vi "Add Record.vi"(8 "Error In (no error)":errorcluster, 10 "Data":variant, 11 "DB Operator in":refnum<class "DB Operator.lvclass">) -> (0 "Error Out":errorcluster, 3 "DB Operator out":refnum<class "DB Operator.lvclass">)   [LabVIEW 2023, in "DB Operator.lvclass"]
uses:
  DB Operator.lvclass
  Ctrls/DB Controls/Category.ctl
  Ctrls/DB Controls/Cycle.ctl
  Ctrls/DB Controls/Saving Goal.ctl
  Ctrls/DB Controls/Saving.ctl
  Ctrls/DB Controls/Subcategory.ctl
  Ctrls/DB Controls/Transaction.ctl
  DB Operator.lvclass/DB Operator.ctl
  <vilib>/Utility/Data Type/NI_Data Type.lvlib
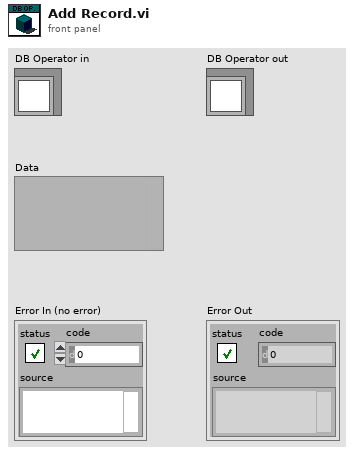
[diagram p1: front panel]
types:
  T1 = typedef "DB Operator.lvclass/Category.ctl" = cluster{"ID":u32, "Name":string}
  T2 = typedef "DB Operator.lvclass/Cycle.ctl" = cluster{"ID":u32, "Name":string, "Day of Month":u8, "Description":string}
  T3 = typedef "DB Operator.lvclass/Saving Goal.ctl" = cluster{"ID":u64, "Is Active":bool, "Name":string, "Current Value":dbl, "Target Value":dbl, "Date of Entry":timestamp, "Due Date":timestamp, "Last Update":timestamp, "Description":string}
  T4 = typedef "DB Operator.lvclass/Saving.ctl" = cluster{"ID":u64, "Value":dbl, "Date of Entry":timestamp, "Saving Goal":u32, "Description":string}
  T5 = typedef "DB Operator.lvclass/Subcategory.ctl" = cluster{"ID":u32, "Name":string, "Category":u32}
  T6 = typedef "DB Operator.lvclass/Transaction.ctl" = cluster{"ID":u64, "Name":string, "Is Income":bool, "Value":dbl, "Amount":dbl, "Total":dbl, "Date of Entry":timestamp, "Date":timestamp, "Last Update":timestamp, "Category":u32, "Subcategory":u32, "Cycle":u32, "Description":string}
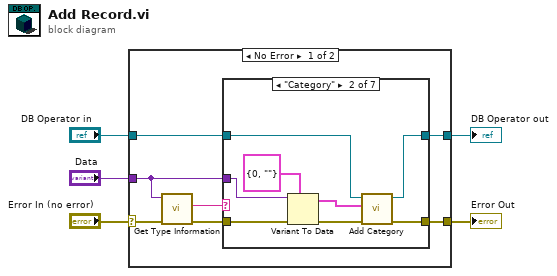
[diagram p0: block diagram]
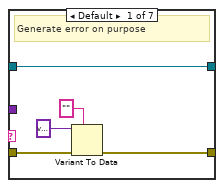
[diagram p2: hidden frame]
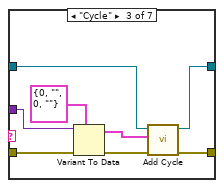
[diagram p3: hidden frame]
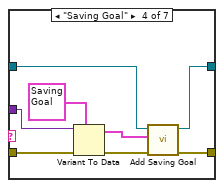
[diagram p4: hidden frame]
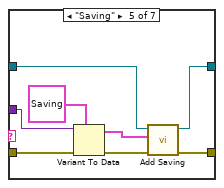
[diagram p5: hidden frame]
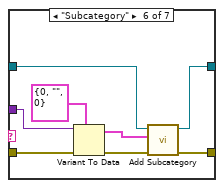
[diagram p6: hidden frame]
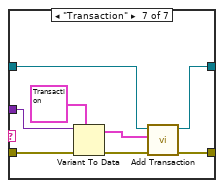
[diagram p7: hidden frame]
diagram:
  n1 = case shown="No Error" "Error In (no error)" {
    selector: "Error In (no error)" -> [w12 w67]
    tunnel: [w7 w67] -> w4
    tunnel: [w6 w66] -> w2
    tunnel: "DB Operator in" -> [w8 w66]
    tunnel: "Data" -> [w9 _]
    frame No Error {
      n2 = call <vilib>:"Get Type Information.vi"("error in (no error)"=w12, "variant"=w9) -> ("error out"=w10:errorcluster, "name"=w11:string)  [unwired: 5 in, 3 out]
      n3 = case shown="\"Category\"" w11 {
        tunnel: w10 -> [w16 w25 w33 w41 w49 w57 w65]
        tunnel: w9 -> [_ w23 w31 w39 w47 w55 w63]
        tunnel: w8 -> [w17 w20 w28 w36 w44 w52 w60]
        tunnel: [w13 w19 w27 w35 w43 w51 w59] -> w7
        tunnel: [w17 w18 w26 w34 w42 w50 w58] -> w6
        frame Default {
          # "Generate error on purpose"
          n4 = Variant To Data(error in=w16, type="", Variant=variant ("variant")) -> (error out=w13:errorcluster)  [unwired: 1 out]
        }
        frame "Category" {
          n5 = Variant To Data(error in=w25, type=T1 {"ID"=0, "Name"=""} ("Category"), Variant=w23) -> (data=w21:T1, error out=w22:errorcluster)
          n6 = call-dynamic "Add Category.vi"("Error In (no error)"=w22, "Category"=w21, "DB Operator In"=w20) -> ("Error Out"=w19:errorcluster, "DB Operator Out"=w18:refnum<class "DB Operator.lvclass">)  [unwired: 7 in]
        }
        frame "Cycle" {
          n7 = Variant To Data(error in=w33, type=T2 {"ID"=0, "Name"="", "Day of Month"=0, "Description"=""} ("Cycle"), Variant=w31) -> (data=w29:T2, error out=w30:errorcluster)
          n8 = call-dynamic "Add Cycle.vi"("Error In (no error)"=w30, "Cycle"=w29, "DB Operator In"=w28) -> ("Error Out"=w27:errorcluster, "DB Operator Out"=w26:refnum<class "DB Operator.lvclass">)  [unwired: 7 in]
        }
        frame "Saving Goal" {
          n9 = Variant To Data(error in=w41, type=T3 {"ID"=0, "Is Active"=FALSE, "Name"="", "Current Value"=0.0, "Target Value"=0.0, "Date of Entry"=timestamp(0 s since 1904-01-01), "Due Date"=timestamp(0 s since 1904-01-01), "Last Update"=timestamp(0 s since 1904-01-01), "Description"=""} ("Saving Goal"), Variant=w39) -> (data=w37:T3, error out=w38:errorcluster)
          n10 = call-dynamic "Add Saving Goal.vi"("Error In (no error)"=w38, "Saving Goal"=w37, "DB Operator In"=w36) -> ("Error Out"=w35:errorcluster, "DB Operator Out"=w34:refnum<class "DB Operator.lvclass">)  [unwired: 7 in]
        }
        frame "Saving" {
          n11 = Variant To Data(error in=w49, type=T4 {"ID"=0, "Value"=0.0, "Date of Entry"=timestamp(0 s since 1904-01-01), "Saving Goal"=0, "Description"=""} ("Saving"), Variant=w47) -> (data=w45:T4, error out=w46:errorcluster)
          n12 = call-dynamic "Add Saving.vi"("Error In (no error)"=w46, "Saving"=w45, "DB Operator In"=w44) -> ("Error Out"=w43:errorcluster, "DB Operator Out"=w42:refnum<class "DB Operator.lvclass">)  [unwired: 7 in]
        }
        frame "Subcategory" {
          n13 = Variant To Data(error in=w57, type=T5 {"ID"=0, "Name"="", "Category"=0} ("Subcategory"), Variant=w55) -> (data=w53:T5, error out=w54:errorcluster)
          n14 = call-dynamic "Add Subcategory.vi"("Error In (no error)"=w54, "Subcategory"=w53, "DB Operator In"=w52) -> ("Error Out"=w51:errorcluster, "DB Operator Out"=w50:refnum<class "DB Operator.lvclass">)  [unwired: 7 in]
        }
        frame "Transaction" {
          n15 = Variant To Data(error in=w65, type=T6 {"ID"=0, "Name"="", "Is Income"=FALSE, "Value"=0.0, "Amount"=0.0, "Total"=0.0, "Date of Entry"=timestamp(0 s since 1904-01-01), "Date"=timestamp(0 s since 1904-01-01), "Last Update"=timestamp(0 s since 1904-01-01), "Category"=0, "Subcategory"=0, "Cycle"=0, "Description"=""} ("Transaction"), Variant=w63) -> (data=w61:T6, error out=w62:errorcluster)
          n16 = call-dynamic "Add Transaction.vi"("Error In (no error)"=w62, "Transaction"=w61, "DB Operator In"=w60) -> ("Error Out"=w59:errorcluster, "DB Operator Out"=w58:refnum<class "DB Operator.lvclass">)  [unwired: 7 in]
        }
      }
    }
    frame Error {
    }
  }
  "Error Out" <- w4
  "DB Operator out" <- w2
